vi "finalize initialization.vi"(8 "error in":errorcluster, 10 "configuration in":refnum<class "control module configuration.lvclass">, 11 "fixed channel runtime in":refnum<class "control module runtime.lvclass">) -> (0 "error out":errorcluster, 3 "fixed channel runtime out":refnum<class "control module runtime.lvclass">)   [LabVIEW 2013, in "control module runtime.lvclass"]
uses:
  control module runtime.lvclass
  configuration/control module configuration.lvclass
  configuration/control module configuration.lvclass/control module configuration.ctl
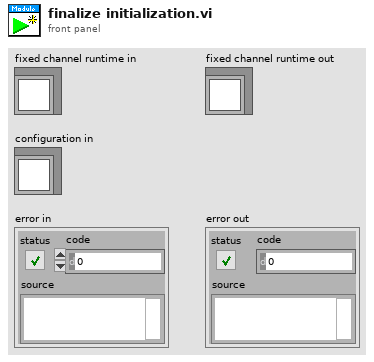
[diagram p1: front panel]
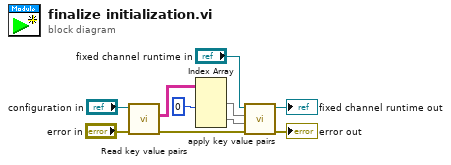
[diagram p0: block diagram]
diagram:
  n1 = call "Read key value pairs.vi"("error in"="error in", "fixed channel configuration in"="configuration in") -> ("error out"=w4:errorcluster, "key value pairs"=w10:string[][])  [unwired: 7 in, 1 out]
  n2 = Index Array(array=w10, index (col) #1=0 ("disabled index (col)")) -> (element #1=w2:string[], element #2=w1:string[])  [unwired: 3 in]
  n3 = call-dynamic "apply key value pairs.vi"("error in"=w4, "values"=w1, "keys"=w2, "fixed channel runtime in"="fixed channel runtime in") -> ("error out"=→"error out":errorcluster, "fixed channel runtime out"=→"fixed channel runtime out":refnum<class "control module runtime.lvclass">)  [unwired: 6 in]
